vi "Plot Control.vi"(8 "Data":dbl[][](array[numeric]), 9 "Rate Selection":u16, 10 "Temperature Selection":u16, 11 "Flow Selection":u16) -> (0 "SUR / HUR Plot":cluster{"Array out":dbl[], "Array out":dbl[]}, 1 "Power Plot":cluster{"Array out":dbl[], "Array out":dbl[]}[](array[cluster]), 2 "Temperature Plot":cluster{"Array out":dbl[], "Array out":dbl[]}[](array[cluster]), 3 "Flow Plot":cluster{"Array out":dbl[], "Array out":dbl[]})   [LabVIEW 2019]
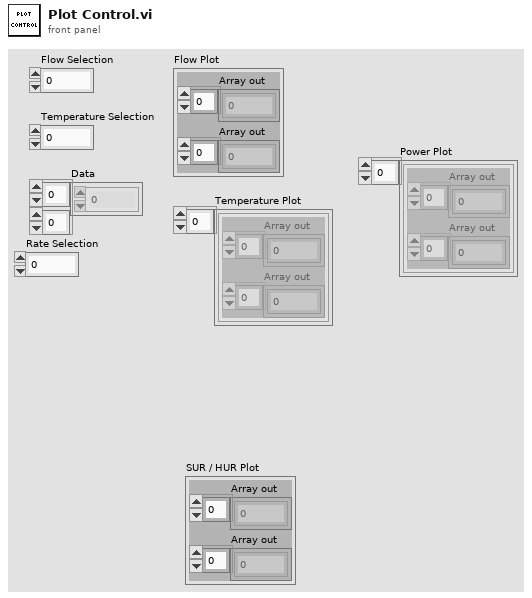
[diagram p1: front panel]
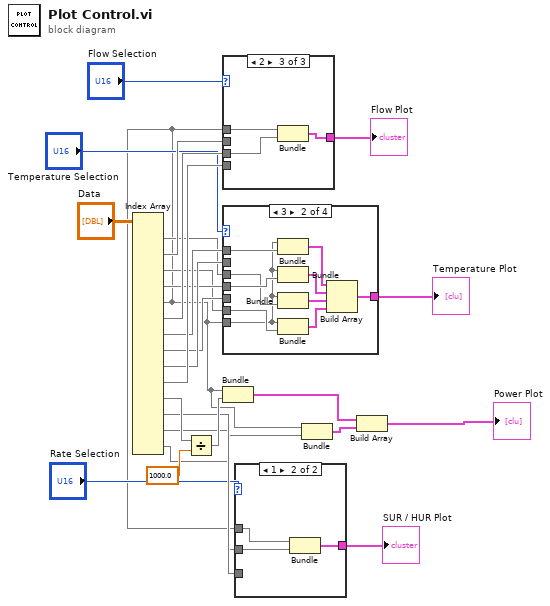
[diagram p0: block diagram]
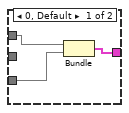
[diagram p2: hidden frame]
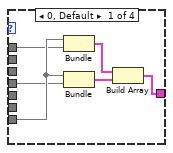
[diagram p3: hidden frame]
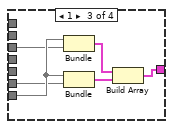
[diagram p4: hidden frame]
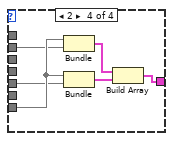
[diagram p5: hidden frame]
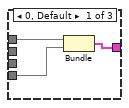
[diagram p6: hidden frame]
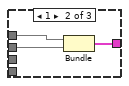
[diagram p7: hidden frame]
diagram:
  n1 = Index Array(array="Data") -> (element #1=w17:dbl[], element #2=w18:dbl[], element #3=w19:dbl[], element #4=w20:dbl[], element #5=w5:dbl[], element #6=w21:dbl[], element #7=w22:dbl[], element #8=w23:dbl[], element #9=w24:dbl[], element #10=w25:dbl[], element #11=w11:dbl[], element #12=w8:dbl[], element #13=w7:dbl[], element #14=w4:dbl[])  [unwired: 28 in]
  n2 = Divide(x=w11, y=1000.0) -> (x/y=w10:dbl[])
  n3 = case shown="2" "Flow Selection" {
    tunnel: w5 -> [w29 w32 w35]
    tunnel: w25 -> [w28 _ _]
    tunnel: [w27 w31 w34] -> w15
    tunnel: w21 -> [_ _ w33]
    tunnel: w18 -> [_ w30 _]
    frame 0, Default {
      n4 = Bundle("Data"=w29, "Data"=w28) -> (w27:cluster{"Data":dbl[], "Data":dbl[]})  [unwired: 1 in]
    }
    frame 1 {
      n5 = Bundle("Data"=w32, "Data"=w30) -> (w31:cluster{"Data":dbl[], "Data":dbl[]})  [unwired: 1 in]
    }
    frame 2 {
      n6 = Bundle("Data"=w35, "Data"=w33) -> (w34:cluster{"Data":dbl[], "Data":dbl[]})  [unwired: 1 in]
    }
  }
  "Flow Plot" <- w15
  n7 = case shown="3" "Temperature Selection" {
    tunnel: w5 -> [w41 w42 w56 w63]
    tunnel: w20 -> [w36 w48 _ _]
    tunnel: w22 -> [w37 w49 _ _]
    tunnel: [w38 w50 w57 w60] -> w16
    tunnel: w17 -> [_ w46 w53 _]
    tunnel: w19 -> [_ w45 w52 _]
    tunnel: w23 -> [_ _ _ w59]
    tunnel: w24 -> [_ _ _ w58]
    frame 0, Default {
      n8 = Bundle("Data"=w41, "Data"=w37) -> (w40:cluster{"Data":dbl[], "Data":dbl[]})  [unwired: 1 in]
      n9 = Bundle("Data"=w41, "Data"=w36) -> (w39:cluster{"Data":dbl[], "Data":dbl[]})  [unwired: 1 in]
      n10 = Build Array(w40, w39) -> (w38:cluster{"Data":dbl[], "Data":dbl[]}[])
    }
    frame 3 {
      n11 = Bundle("Data"=w42, "Data"=w49) -> (w51:cluster{"Data":dbl[], "Data":dbl[]})  [unwired: 1 in]
      n12 = Bundle("Data"=w42, "Data"=w48) -> (w47:cluster{"Data":dbl[], "Data":dbl[]})  [unwired: 1 in]
      n13 = Bundle("Data"=w42, "Data"=w46) -> (w44:cluster{"Data":dbl[], "Data":dbl[]})  [unwired: 1 in]
      n14 = Bundle("Data"=w42, "Data"=w45) -> (w43:cluster{"Data":dbl[], "Data":dbl[]})  [unwired: 1 in]
      n15 = Build Array(w51, w47, w44, w43) -> (w50:cluster{"Data":dbl[], "Data":dbl[]}[])
    }
    frame 1 {
      n16 = Bundle("Data"=w56, "Data"=w53) -> (w55:cluster{"Data":dbl[], "Data":dbl[]})  [unwired: 1 in]
      n17 = Bundle("Data"=w56, "Data"=w52) -> (w54:cluster{"Data":dbl[], "Data":dbl[]})  [unwired: 1 in]
      n18 = Build Array(w55, w54) -> (w57:cluster{"Data":dbl[], "Data":dbl[]}[])
    }
    frame 2 {
      n19 = Bundle("Data"=w63, "Data"=w58) -> (w62:cluster{"Data":dbl[], "Data":dbl[]})  [unwired: 1 in]
      n20 = Bundle("Data"=w63, "Data"=w59) -> (w61:cluster{"Data":dbl[], "Data":dbl[]})  [unwired: 1 in]
      n21 = Build Array(w62, w61) -> (w60:cluster{"Data":dbl[], "Data":dbl[]}[])
    }
  }
  "Temperature Plot" <- w16
  n22 = Bundle("Data"=w5, w10) -> (w3:cluster{"Data":dbl[], dbl[]})  [unwired: 1 in]
  n23 = case shown="1" "Rate Selection" {
    tunnel: w8 -> [w66 _]
    tunnel: [w65 w69] -> w9
    tunnel: w7 -> [_ w68]
    tunnel: w5 -> [w64 w67]
    frame 0, Default {
      n24 = Bundle("Data"=w64, "Data"=w66) -> (w65:cluster{"Data":dbl[], "Data":dbl[]})  [unwired: 1 in]
    }
    frame 1 {
      n25 = Bundle("Data"=w67, "Data"=w68) -> (w69:cluster{"Data":dbl[], "Data":dbl[]})  [unwired: 1 in]
    }
  }
  "SUR / HUR Plot" <- w9
  n26 = Bundle("Data"=w5, "Data"=w4) -> (w2:cluster{"Data":dbl[], "Data":dbl[]})  [unwired: 1 in]
  n27 = Build Array(w3, w2) -> (→"Power Plot":cluster{"Data":dbl[], "Data":dbl[]}[])
